vi "sv_Peaks to Phases.vi"(0 "peaks":cluster{"frequency":dbl, "value":dbl}[](array[cluster]) {"value" format="%.2f"; "frequency" format="%.2f"}, 1 "phase [radians]":cluster{"f0":dbl, "df":dbl, "phase":dbl[]} {"phase" format="%.2f"; "df" format="%.2f"; "f0" format="%.2f"}, 5 "error in":errorcluster, 6 "desired units":T2, 8 "frequency range string":string) -> (11 "average group delay":dbl format="%.2f", 12 "unit labels":T1, 13 "maximum phase deviation":dbl format="%.2f", 14 "frequencies [Hz]":dbl[](array[numeric]) format="%.2f", 15 "phases":dbl[](array[numeric]) format="%.2f", 16 "multitone phases":cluster{"frequency":dbl, "phase":dbl}[](array[cluster]) {"phase" format="%.2f"; "frequency" format="%.2f"}, 17 "phases":cluster{"frequencies":dbl[], "phases":dbl[]}[](array[cluster]) {"phases" format="%.2f"; "frequencies" format="%.2f"}, 18 "phase deviation":cluster{"frequencies":dbl[], "phases":dbl[]} {"phases" format="%.2f"; "frequencies" format="%.2f"}, 19 "error out":errorcluster)   [LabVIEW 2017, in "SoundVib_Distortion.lvlib"]
uses:
  <vilib>/addons/Sound and Vibration/svt_Distortion/SoundVib_Distortion.lvlib
  <vilib>/Analysis/NI_AALPro.lvlib
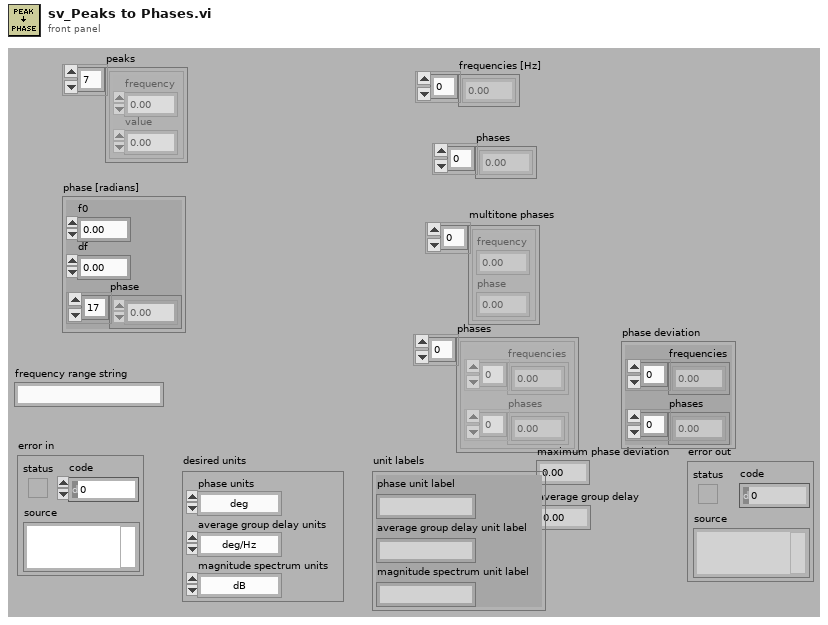
[diagram p1: front panel]
types:
  T1 = cluster{"phase unit label":string, "average group delay unit label":string, "magnitude spectrum unit label":string}
  T2 = cluster{"phase units":enum16{"deg", "rad"}, "average group delay units":enum16{"deg/Hz", "s"}, "magnitude spectrum units":enum16{"dB", "linear"}}
  T3 = cluster{string, string, "unit label (phase)":string}
  T4 = cluster{"unit label (phase)":string, "unit label (phase)":string, "unit label (phase)":string}
  T5 = enum16{"even-spaced multitone", "square wave", "test signal not recognized"}
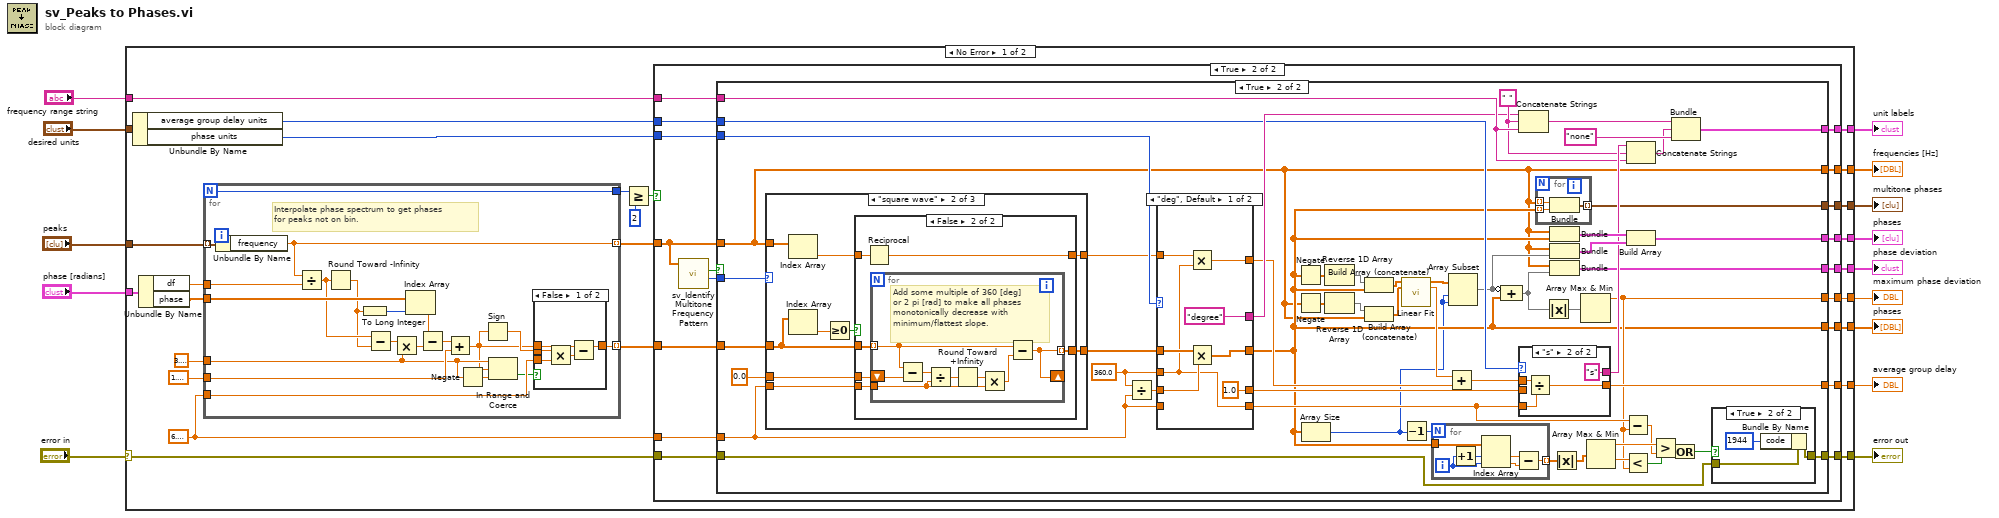
[diagram p0: block diagram]
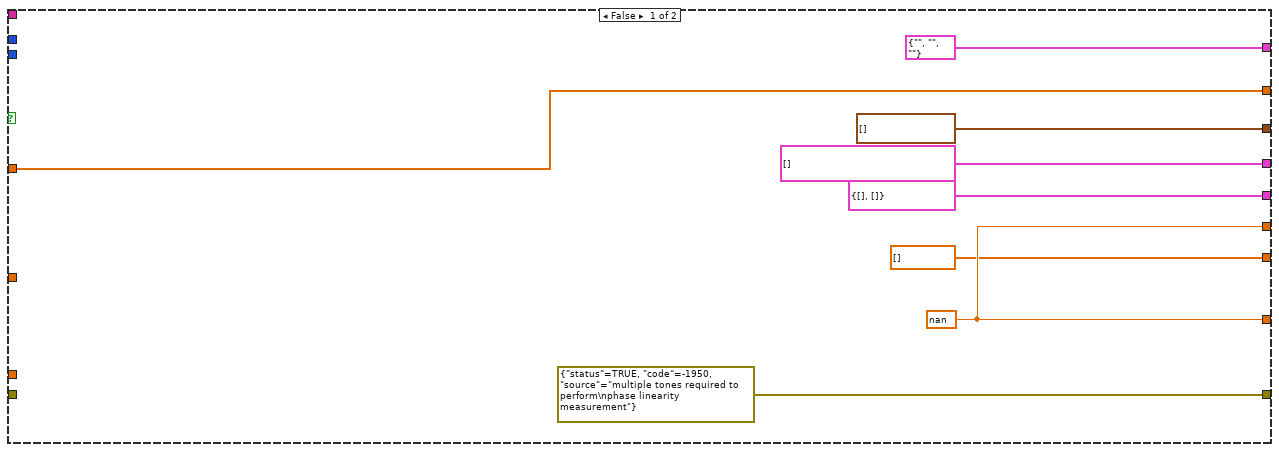
[diagram p2: hidden frame]
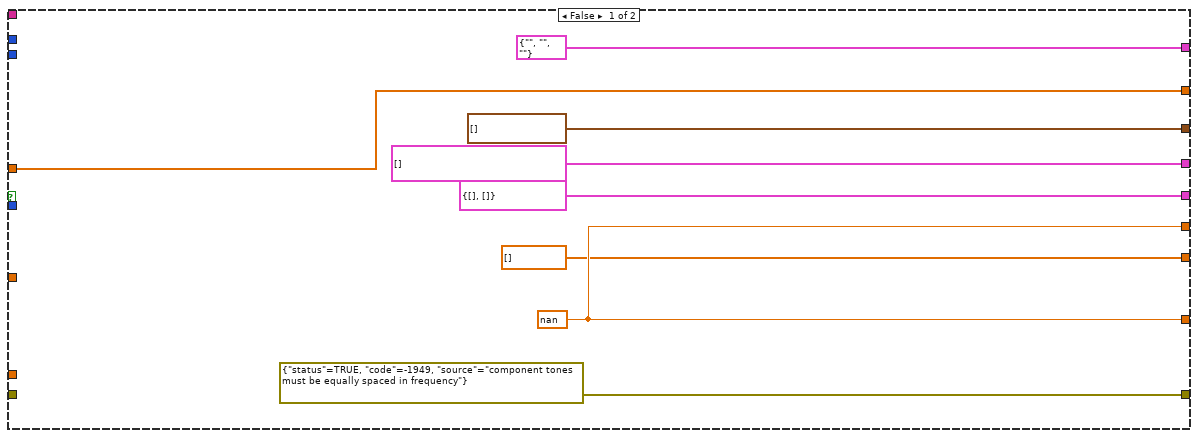
[diagram p3: hidden frame]
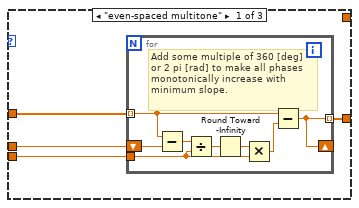
[diagram p5: hidden frame]
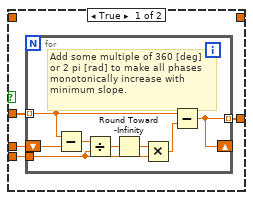
[diagram p6: hidden frame]
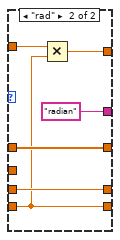
[diagram p8: hidden frame]
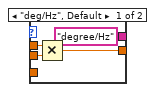
[diagram p9: hidden frame]
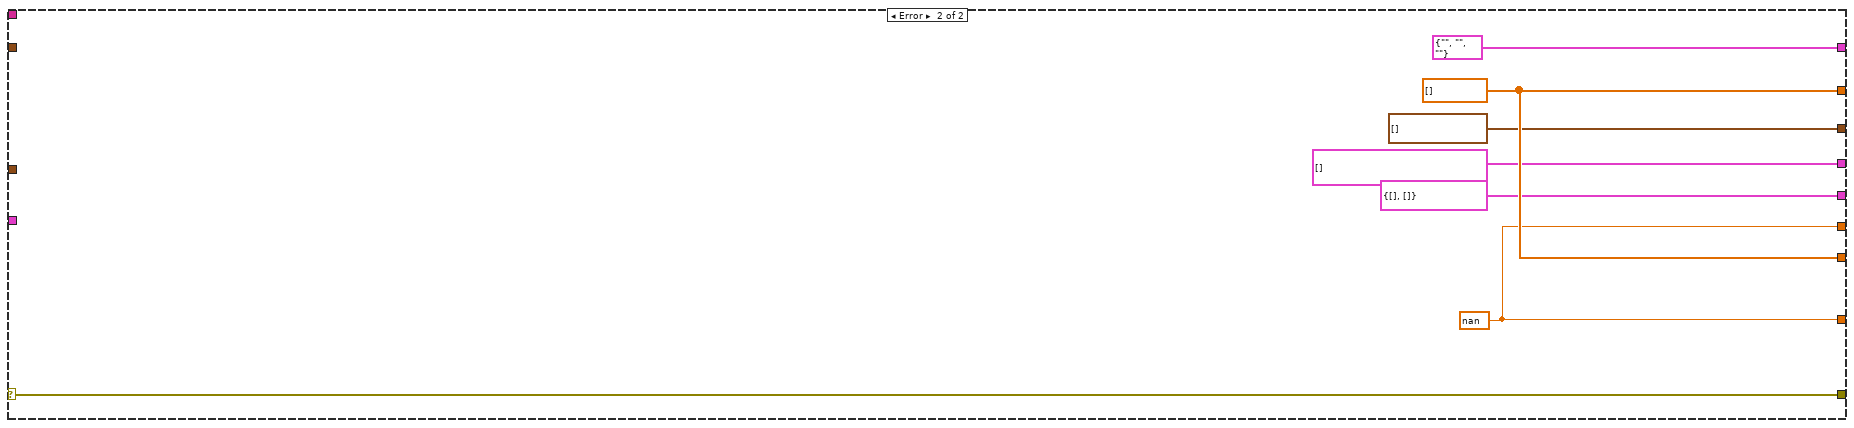
[diagram p11: hidden frame]
diagram:
  n1 = case shown="No Error" "error in" {
    selector: "error in" -> [w25 w244]
    tunnel: [w26 w243] -> w14
    tunnel: "peaks" -> [w40 _]
    tunnel: [w24 w243] -> w12
    tunnel: "phase [radians]" -> [w38 _]
    tunnel: [w28 cluster{"frequency":dbl, dbl}[] []] -> w10
    tunnel: [w33 w242] -> w9
    tunnel: [w36 cluster{dbl[], "Best Linear Fit":dbl[]}[] []] -> w8
    tunnel: [w35 w242] -> w7
    tunnel: [w23 w244] -> w5
    tunnel: "desired units" -> [w34 _]
    tunnel: [w32 T4 {"unit label (phase)"="", "unit label (phase)"="", "unit label (phase)"=""}] -> w3
    tunnel: "frequency range string" -> [w31 _]
    tunnel: [w15 cluster{dbl[], dbl[]} {[], []}] -> w1
    frame No Error {
      w16 = 6.283185307179586
      n2 = Unbundle By Name(w34) -> ("average group delay units"=w29:enum16{"deg/Hz", "s"}, "phase units"=w27:enum16{"deg", "rad"})
      n3 = Unbundle By Name(w38) -> ("df"=w37:dbl, "phase"=w39:dbl[])
      n4 = for {
        N -> [w220]
        tunnel: w40 -> [w231] mode=indexing
        tunnel: w39 -> [w230]
        tunnel: w37 -> [w228]
        tunnel: [w212] -> w30 mode=indexing
        tunnel: [w221] -> w21 mode=indexing
        tunnel: 3.141592653589793 -> [w217]
        tunnel: [w220] -> w20
        tunnel: 1.5707963267948966 -> [w219]
        tunnel: w16 -> [w215]
        # "Interpolate phase spectrum to get phases\nfor peaks not on bin."
        n5 = Unbundle By Name(w231) -> ("frequency"=w221:dbl)
        n6 = Divide(x=w221, y=w228) -> (x/y=w227:dbl)
        n7 = Round Toward -Infinity(1:w227) -> (0:w226:dbl)
        n8 = To Long Integer(number=w226) -> (32bit integer=w229:i32)
        n9 = Subtract(x=w227, y=w226) -> (x-y=w225:dbl)
        n10 = Multiply(x=w225, y=w217) -> (x*y=w223:dbl)
        n11 = Index Array(array=w230, index=w229) -> (element=w224:dbl)
        n12 = Subtract(x=w224, y=w223) -> (x-y=w222:dbl)
        n13 = Add(x=w222, y=w219) -> (x+y=w213:dbl)
        n14 = Negate(x=w217) -> (-x=w218:dbl)
        n15 = Sign(1:w213) -> (0:w216:dbl)
        n16 = In Range and Coerce(upper limit=w217, x=w213, lower limit=w218) -> (In Range?=w214:bool)  [unwired: 1 out]
        n17 = case shown="False" w214 {
          tunnel: w216 -> [w236 _]
          tunnel: w215 -> [w235 _]
          tunnel: [w233 w237] -> w212
          tunnel: w213 -> [w232 w237]
          frame False {
            n18 = Multiply(x=w236, y=w235) -> (x*y=w234:dbl)
            n19 = Subtract(x=w232, y=w234) -> (x-y=w233:dbl)
          }
          frame True {
          }
        }
      }
      n20 = Greater Or Equal?(x=w20, y=2) -> (x >= y?=w18:bool)
      n21 = case shown="True" w18 {
        tunnel: [cluster{dbl[], "Best Linear Fit":dbl[]}[] [] w66] -> w36
        tunnel: [w44 w65] -> w35
        tunnel: [w44 w64] -> w33
        tunnel: [T3 {"", "", "unit label (phase)"=""} w63] -> w32
        tunnel: w31 -> [_ w62]
        tunnel: w30 -> [_ w61]
        tunnel: w29 -> [_ w60]
        tunnel: [cluster{"frequency":dbl, dbl}[] [] w59] -> w28
        tunnel: w27 -> [_ w58]
        tunnel: [dbl[] [] w57] -> w26
        tunnel: w25 -> [_ w56]
        tunnel: [w47 w54] -> w24
        tunnel: [errorcluster {"status"=TRUE, "code"=-1950, "source"="multiple tones required to perform\nphase linearity measurement"} ("error IO") w53] -> w23
        tunnel: w21 -> [w47 w52]
        tunnel: w16 -> [_ w50]
        tunnel: [cluster{dbl[], dbl[]} {[], []} w49] -> w15
        frame False {
          w44 = nan
        }
        frame True {
          n22 = call <vilib>:"sv_Identify Multitone Frequency Pattern.vi"("frequencies"=w52) -> ("test signal"=w51:T5, "valid test signal"=w55:bool)  [unwired: 9 in]
          n23 = case shown="True" w55 {
            tunnel: [cluster{dbl[], "Best Linear Fit":dbl[]}[] [] w125] -> w66
            tunnel: [w70 w93] -> w65
            tunnel: [w70 w124] -> w64
            tunnel: [T3 {"", "", "unit label (phase)"=""} w122] -> w63
            tunnel: w62 -> [_ w119]
            tunnel: w61 -> [_ w117]
            tunnel: w60 -> [_ w112]
            tunnel: [cluster{"frequency":dbl, dbl}[] [] w111] -> w59
            tunnel: w58 -> [_ w110]
            tunnel: [dbl[] [] w85] -> w57
            tunnel: w52 -> [w74 w76]
            tunnel: w56 -> [_ w91]
            tunnel: [w74 w76] -> w54
            tunnel: [errorcluster {"status"=TRUE, "code"=-1949, "source"="component tones must be equally spaced in frequency"} ("error IO") w92] -> w53
            tunnel: w51 -> [_ w106]
            tunnel: w50 -> [_ w101]
            tunnel: [cluster{dbl[], dbl[]} {[], []} w75] -> w49
            frame False {
              w70 = nan
            }
            frame True {
              w108 = 360.0
              w118 = " " ("string")
              n24 = case shown="\"square wave\"" w106 {
                tunnel: w117 -> [w139 w156 w186]
                tunnel: 0.0 -> [w142 w159 _]
                tunnel: [w141 w158 w186] -> w113
                tunnel: w101 -> [w140 w157 _]
                tunnel: w76 -> [_ w154 _]
                tunnel: [_ w152 _] -> w103
                frame "even-spaced multitone" {
                  n25 = for {
                    tunnel: w139 -> [w143] mode=indexing
                    tunnel: [w144] -> w141 mode=indexing
                    shift-right: [w144] -> _
                    shift-left: w142 -> [w146]
                    tunnel: w140 -> [w145]
                    # "Add some multiple of 360 [deg]\nor 2 pi [rad] to make all phases \nmonotonically increase with \nminimum slope."
                    n26 = Subtract(x=w143, y=w146) -> (x-y=w147:dbl)
                    n27 = Divide(x=w147, y=w145) -> (x/y=w148:dbl)
                    n28 = Round Toward -Infinity(1:w148) -> (0:w149:dbl)
                    n29 = Multiply(x=w149, y=w145) -> (x*y=w150:dbl)
                    n30 = Subtract(x=w143, y=w150) -> (x-y=w144:dbl)
                  }
                }
                frame "square wave" {
                  n31 = Index Array(array=w154) -> (element=w153:dbl)  [unwired: 1 in]
                  n32 = Index Array(array=w156) -> (element=w151:dbl)  [unwired: 1 in]
                  n33 = Greater Or Equal To 0?(x=w151) -> (x >= 0?=w155:bool)
                  n34 = case shown="False" w155 {
                    tunnel: w159 -> [w163 w177]
                    tunnel: [w162 w176] -> w158
                    tunnel: w157 -> [w161 w175]
                    tunnel: w156 -> [w160 w174]
                    tunnel: w153 -> [_ w173]
                    tunnel: [_ w172] -> w152
                    frame True {
                      n35 = for {
                        tunnel: w160 -> [w164] mode=indexing
                        tunnel: [w165] -> w162 mode=indexing
                        shift-right: [w165] -> _
                        shift-left: w163 -> [w167]
                        tunnel: w161 -> [w166]
                        # "Add some multiple of 360 [deg]\nor 2 pi [rad] to make all phases \nmonotonically increase with \nminimum slope."
                        n36 = Subtract(x=w164, y=w167) -> (x-y=w168:dbl)
                        n37 = Divide(x=w168, y=w166) -> (x/y=w169:dbl)
                        n38 = Round Toward -Infinity(1:w169) -> (0:w170:dbl)
                        n39 = Multiply(x=w170, y=w166) -> (x*y=w171:dbl)
                        n40 = Subtract(x=w164, y=w171) -> (x-y=w165:dbl)
                      }
                    }
                    frame False {
                      n41 = Reciprocal(x=w173) -> (1/x=w172:dbl)
                      n42 = for {
                        tunnel: w174 -> [w178] mode=indexing
                        tunnel: [w179] -> w176 mode=indexing
                        shift-right: [w179] -> _
                        shift-left: w177 -> [w181]
                        tunnel: w175 -> [w180]
                        # "Add some multiple of 360 [deg]\nor 2 pi [rad] to make all phases \nmonotonically decrease with \nminimum/flattest slope."
                        n43 = Subtract(x=w178, y=w181) -> (x-y=w182:dbl)
                        n44 = Divide(x=w182, y=w180) -> (x/y=w183:dbl)
                        n45 = Round Toward +Infinity(x=w183) -> (ceil(x): smallest int >= x=w184:dbl)
                        n46 = Multiply(x=w184, y=w180) -> (x*y=w185:dbl)
                        n47 = Subtract(x=w178, y=w185) -> (x-y=w179:dbl)
                      }
                    }
                  }
                }
                frame "test signal not recognized", Default {
                }
              }
              n48 = Divide(x=w108, y=w101) -> (x/y=w109:dbl)
              n49 = case shown="\"deg\", Default" w110 {
                tunnel: w113 -> [w194 w201]
                tunnel: [w197 w201] -> w85
                tunnel: w109 -> [w193 w203]
                tunnel: [1.0 w203] -> w114
                tunnel: w101 -> [_ w199]
                tunnel: ["degree" ("unit label (phase)") "radian" ("unit label (phase)")] -> w115
                tunnel: [w191 w199] -> w96
                tunnel: w108 -> [w191 _]
                tunnel: w103 -> [w192 w200]
                tunnel: [w190 w198] -> w102
                frame "deg", Default {
                  n50 = Multiply(x=w192, y=w191) -> (x*y=w190:dbl)
                  n51 = Multiply(x=w194, y=w193) -> (x*y=w197:dbl[])
                }
                frame "rad" {
                  n52 = Multiply(x=w200, y=w199) -> (x*y=w198:dbl)
                }
              }
              n53 = Negate(x=w85) -> (-x=w87:dbl[])
              n54 = Negate(x=w76) -> (-x=w82:dbl[])
              n55 = Array Size(array=w85) -> (size(s)=w78:i32)
              n56 = Reverse 1D Array(array=w87) -> (reversed array=w86:dbl[])
              n57 = Reverse 1D Array(array=w82) -> (reversed array=w83:dbl[])
              n58 = Build Array (concatenate)(w86, w85) -> (w84:dbl[])
              n59 = Build Array (concatenate)(w83, w76) -> (w81:dbl[])
              n60 = call <vilib>:"Linear Fit.vi"("Y"=w84, "X"=w81) -> ("Best Linear Fit"=w80:dbl[], "slope"=w105:dbl)  [unwired: 9 in, 3 out]
              n61 = Decrement(x=w78) -> (x-1=w100:i32)
              n62 = for {
                N: w100 -> [_]
                tunnel: w85 -> [w138]
                tunnel: [w133] -> w99 mode=indexing
                i -> [w136]
                n63 = Increment(x=w136) -> (x+1=w137:i32)
                n64 = Index Array(array=w138, index #1=w137, index #2=w136) -> (element #1=w134:dbl, element #2=w135:dbl)
                n65 = Subtract(x=w134, y=w135) -> (x-y=w133:dbl)
              }
              n66 = Add(x=w105, y=w102) -> (x+y=w104:dbl)
              n67 = Array Subset(array=w80, index=w78, length=w78) -> (w79:dbl[])
              n68 = Compound Arithmetic op=ADD(invert w79, w85) -> (w77:dbl[])
              n69 = Concatenate Strings(w115, w118, w119) -> (w120:string)
              n70 = case shown="\"s\"" w112 {
                tunnel: w104 -> [w206 w210]
                tunnel: w114 -> [w207 _]
                tunnel: [w205 w209] -> w124
                tunnel: w96 -> [_ w211]
                tunnel: ["degree/Hz" ("unit label (phase)") "s" ("unit label (phase)")] -> w121
                frame "deg/Hz", Default {
                  n71 = Multiply(x=w206, y=w207) -> (x*y=w205:dbl)
                }
                frame "s" {
                  n72 = Divide(x=w210, y=w211) -> (x/y=w209:dbl)
                }
              }
              n73 = for {
                tunnel: [w189] -> w111 mode=indexing
                tunnel: w85 -> [w188] mode=indexing
                tunnel: w76 -> [w187] mode=indexing
                n74 = Bundle("frequency"=w187, w188) -> (w189:cluster{"frequency":dbl, dbl})  [unwired: 1 in]
              }
              n75 = Absolute Value(x=w77) -> (abs(x)=w126:dbl[])
              n76 = Bundle(w76, w85) -> (w128:cluster{dbl[], dbl[]})  [unwired: 1 in]
              n77 = Bundle(w76, w79) -> (w127:cluster{dbl[], dbl[]})  [unwired: 1 in]
              n78 = Bundle(w76, w77) -> (w75:cluster{dbl[], dbl[]})  [unwired: 1 in]
              n79 = Absolute Value(x=w99) -> (abs(x)=w98:dbl[])
              n80 = Array Max & Min(array=w126) -> (max value=w93:dbl)  [unwired: 3 out]
              n81 = Array Max & Min(array=w98) -> (max value=w97:dbl, min value=w95:dbl)  [unwired: 2 out]
              n82 = Subtract(x=w96, y=w93) -> (x-y=w94:dbl)
              n83 = Less?(x=w95, y=w93) -> (x < y?=w89:bool)
              n84 = Concatenate Strings(w121, w118, w119) -> (w107:string)
              n85 = Build Array(w128, w127) -> (w125:cluster{dbl[], dbl[]}[])
              n86 = Greater?(x=w97, y=w94) -> (0:w90:bool)
              n87 = Or(x=w90, y=w89) -> (x .or. y?=w88:bool)
              n88 = Bundle(w120, w107, "unit label (phase)"="none") -> (w122:T3)  [unwired: 1 in]
              n89 = case shown="True" w88 {
                tunnel: [w129 w131] -> w92
                tunnel: w91 -> [w129 w132]
                frame False {
                }
                frame True {
                  n90 = Bundle By Name(cluster=w132, "code"=1944) -> (w131:errorcluster)
                }
              }
            }
          }
        }
      }
    }
    frame Error {
      w242 = nan
      w243 = dbl[] []
    }
  }
  "phases" <- w14
  "frequencies [Hz]" <- w12
  "multitone phases" <- w10
  "phases" <- w8
  "maximum phase deviation" <- w7
  "average group delay" <- w9
  "error out" <- w5
  "unit labels" <- w3
  "phase deviation" <- w1
